vi "TDMS Upload Example.vi"() -> ()   [LabVIEW 2024]
doc: "TDMS upload example."
uses:
  Sift API/Sift Client.lvclass
panel:
  in  "Asset Name":string="LabVIEW-TDMS-Example"
  in  "Path":path
  out "Error":errorcluster
  in  "API Key":string
  in  "API URL":string
  # "Instructions\n\n1. Fill in the API URL, API Key, and Organization ID. Visit this URL for more information on authentication\n    https://docs.siftstack.com/docs/api/authentication\n\n2. Select a TDMS file to upload.\n\n3. Run the VI.\n\n3. The VI should run to completetion with no errors. Navigate to the Sift home page and find the \n     asset to see the example data."
  # "Sift TDMS Upload Example"
  # "Run this example to test uploading TDMS files to Sift."
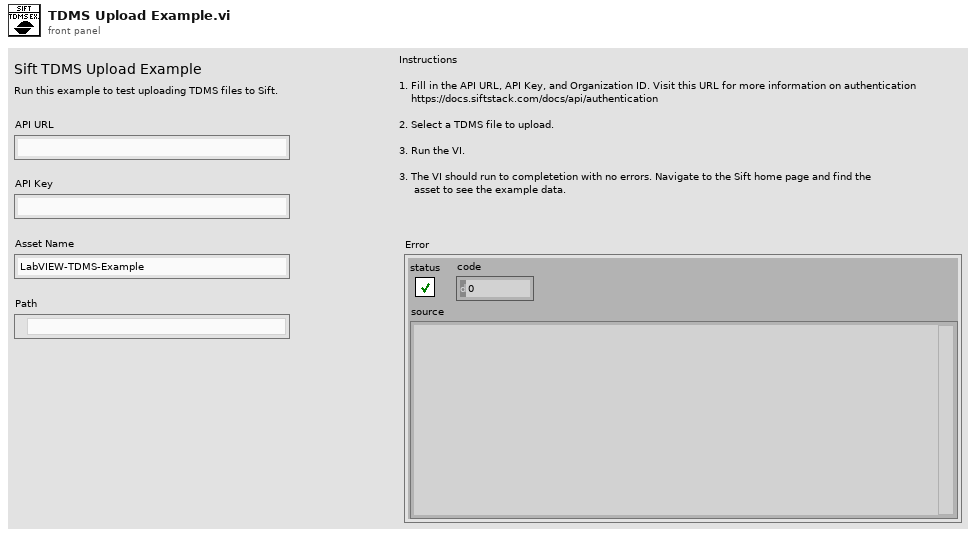
[diagram p1: front panel]
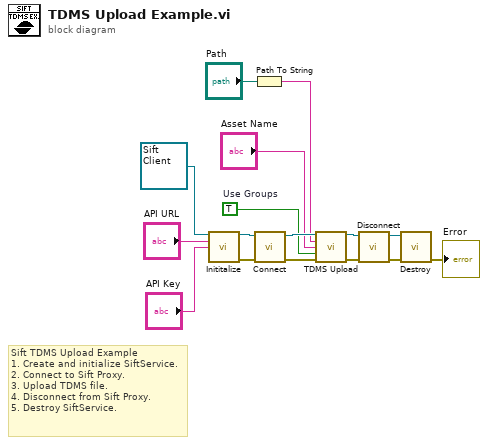
[diagram p0: block diagram]
diagram:
  w2 = TRUE  # Use Groups
  # "Sift TDMS Upload Example\n1. Create and initialize SiftService.\n2. Connect to Sift Proxy.\n3. Upload TDMS file.\n4. Disconnect from Sift Proxy.\n5. Destroy SiftService."
  n1 = call-dynamic "Inititalize.vi"("Sift Client in"=refnum<class "Sift Client.lvclass"> refnum ("Sift Client.lvlib:Sift Client.lvclass"), "API URL"="API URL", "API Key"="API Key") -> ("Sift Client out"=w12:refnum<class "Sift Client.lvclass">, "error out"=w11:errorcluster)  [unwired: 11 in]
  n2 = Path To String(path="Path") -> (string=w1:string)
  n3 = call-dynamic "Connect.vi"("error in (no error)"=w11, "Sift Client in"=w12) -> ("error out"=w9:errorcluster, "Sift Client out"=w10:refnum<class "Sift Client.lvclass">)  [unwired: 7 in, 1 out]
  n4 = call-dynamic "TDMS Upload.vi"("Sift Client in"=w10, "Filepath"=w1, "Asset Name"="Asset Name", "Group Into Components"=w2, "error in (no error)"=w9) -> ("Sift Client out"=w8:refnum<class "Sift Client.lvclass">, "error out"=w7:errorcluster)  [unwired: 9 in]
  n5 = call-dynamic "Disconnect.vi"("error in (no error)"=w7, "Sift Client in"=w8) -> ("error out"=w5:errorcluster, "Sift Client out"=w6:refnum<class "Sift Client.lvclass">)  [unwired: 8 in]
  n6 = call-dynamic "Destroy.vi"("error in (no error)"=w5, "Sift Client in"=w6) -> ("error out"=→"Error":errorcluster)  [unwired: 8 in, 1 out]
